vi "CAN Look Up Channel.vi"(8 "error in (no error)":errorcluster, 10 "FoundChannel":u16, 11 "Parameters":string) -> (0 "error out":errorcluster, 1 "function return":u32, 2 "FoundChannel out":u16, 3 "Parameters out":string)   [LabVIEW 2025, in "PCAN2023.lvlib"]
doc: "Finds a PCAN-Basic channel that matches with the given parameters\n\n\nTPCANStatus __stdcall CAN_LookUpChannel(\n LPSTR Parameters, \n TPCANHandle* FoundChannel);"
uses:
  PCAN2023.lvlib
  x64/PCANBasic.dll
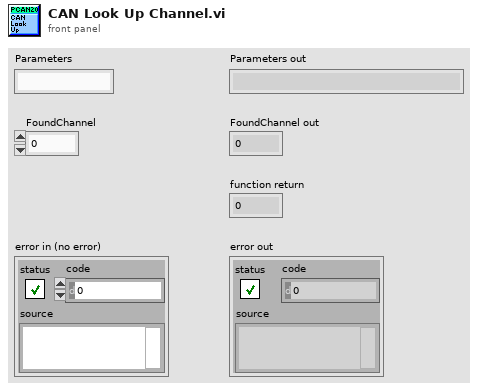
[diagram p1: front panel]
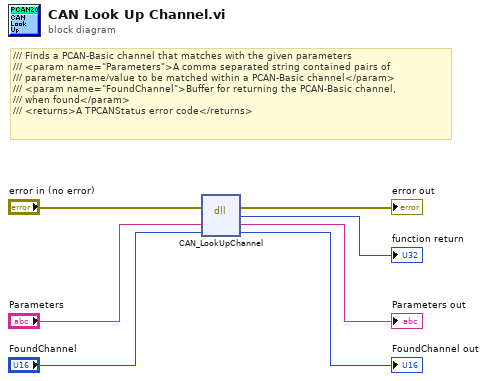
[diagram p0: block diagram]
diagram:
  # "/// Finds a PCAN-Basic channel that matches with the given parameters\n/// <param name=\"Parameters\">A comma separated string contained pairs of \n/// parameter-name/value to be matched within a PCAN-Basic channel</param>\n/// <param name=\"FoundChannel\">Buffer for returning the PCAN-Basic channel, \n/// when found</param>\n/// <returns>A TPCANStatus error code</returns>"
  n1 = dll-call lib="C:/UTP/LabView/Communication Handle/PCAN2023/x64/PCANBasic.dll" fn="CAN_LookUpChannel"(error in="error in (no error)", "Parameters"="Parameters", "FoundChannel"="FoundChannel") -> (error out=→"error out":errorcluster, "return type"=→"function return":u32, "Parameters"=→"Parameters out":string, "FoundChannel"=→"FoundChannel out":u16)  [unwired: 2 in, 1 out]
